vi "Update.vi"(8 "Index":i32, 9 "Pipe Colors in":u32[](array[colorbox]), 10 "Values in":dbl[](array[numeric]), 11 "Pipe in":T1) -> (1 "Pipe Colors out":u32[](array[colorbox]), 2 "Values out":dbl[](array[numeric]))   [LabVIEW 2022 SP3, in "Pipes.lvlib"]
uses:
  Pipes.lvlib
  Controls/Pipe.ctl
  Controls/Pipe Definition.ctl
  Controls/Token Type.ctl
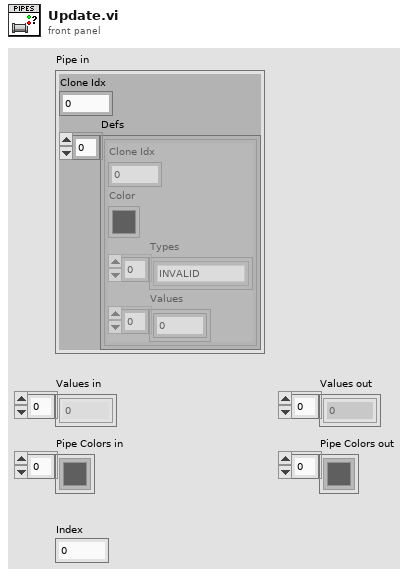
[diagram p1: front panel]
types:
  T1 = typedef "Pipes.lvlib/Pipe.ctl" = cluster{"Clone Idx":i32, "Defs":T2[]}
  T2 = typedef "Pipes.lvlib/Pipe Definition.ctl" = cluster{"Clone Idx":i32, "Color":u32, "Types":T3[], "Values":dbl[]}
  T3 = typedef "Pipes.lvlib/Token Type.ctl" = enum8{"INVALID", "NOT", "AND", "OR", "EE", "NE", "LT", "GT", "LTE", "GTE", "PLUS", "MINUS", "MULTIPLY", "DIVIDE", "MODULUS", "LPAREN", "RPAREN", "LITERAL", "IDENTIFIER", "DEFINITION"}
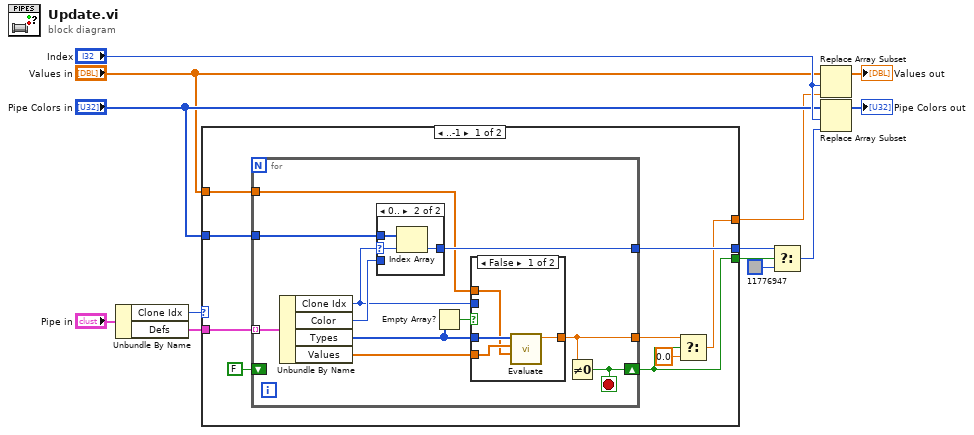
[diagram p0: block diagram]
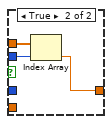
[diagram p3: hidden frame]
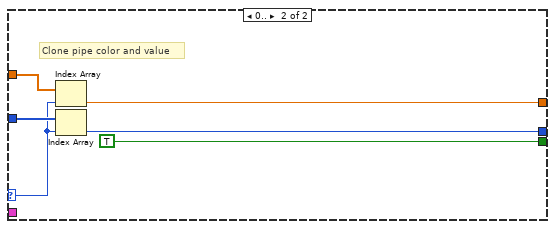
[diagram p4: hidden frame]
diagram:
  n1 = Unbundle By Name("Pipe in") -> ("Clone Idx"=w7:i32, "Defs"=w2:T2[])
  n2 = case shown="..-1" w7 {
    selector: w7 -> [_ w49]
    tunnel: "Pipe Colors in" -> [w21 w50]
    tunnel: "Values in" -> [w19 w48]
    tunnel: [w14 w47] -> w4
    tunnel: [w20 w46] -> w3
    tunnel: w2 -> [w22 _]
    tunnel: [w17 TRUE ("s")] -> w1
    frame ..-1 {
      n3 = for {
        tunnel: w22 -> [w33] mode=indexing
        tunnel: w21 -> [w32]
        tunnel: [w30] -> w20
        tunnel: w19 -> [w26]
        shift-right: [w23] -> w17
        shift-left: FALSE -> [_]
        tunnel: [w24] -> w16
        stop <- w23 stop-if-true
        n4 = Unbundle By Name(w33) -> ("Clone Idx"=w25:i32, "Color"=w31:u32, "Types"=w28:T3[], "Values"=w27:dbl[])
        n5 = case shown="0.." w25 {
          selector: w25 -> [_ w36]
          tunnel: w32 -> [_ w37]
          tunnel: [w34 w35] -> w30
          tunnel: w31 -> [w34 _]
          frame ..-1 {
          }
          frame 0.. {
            n6 = Index Array(array=w37, index=w36) -> (element=w35:u32)
          }
        }
        n7 = Empty Array?(array=w28) -> (empty?=w29:bool)
        n8 = case shown="False" w29 {
          tunnel: w28 -> [w41 _]
          tunnel: w27 -> [w40 _]
          tunnel: w26 -> [w38 w43]
          tunnel: w25 -> [_ w44]
          tunnel: [w39 w42] -> w24
          frame False {
            n9 = call "Evaluate.vi"("Variable Values"=w38, "Values"=w40, "Types"=w41) -> ("Evalulated"=w39:dbl)  [unwired: 8 in]
          }
          frame True {
            n10 = Index Array(array=w43, index=w44) -> (element=w42:dbl)
          }
        }
        n11 = Not Equal To 0?(x=w24) -> (x != 0?=w23:bool)
      }
      n12 = Select(t=w16, s=w17, f=0.0) -> (s? t:f=w14:dbl)
    }
    frame 0.. {
      # "Clone pipe color and value"
      n13 = Index Array(array=w48, index=w49) -> (element=w47:dbl)
      n14 = Index Array(array=w50, index=w49) -> (element=w46:u32)
    }
  }
  n15 = Select(t=w3, s=w1, f=u32 11776947) -> (s? t:f=w10:u32)
  n16 = Replace Array Subset(array="Values in", new element=w4, index="Index") -> (→"Values out":dbl[])
  n17 = Replace Array Subset(array="Pipe Colors in", new element=w10, index="Index") -> (→"Pipe Colors out":u32[])
